vi "SplitLinesByDevice.vi"(8 "error in":errorcluster, 11 "Lines":tag[](array[tag])) -> (0 "error out":errorcluster, 1 "Num lines":i32, 2 "Original indices":i32[][](array[numeric]), 3 "Lines by device":string[](array[string]))   [LabVIEW 2015]
doc: "Splits the input lines into an array of lines where each array element is a flattened (comma-delimited string) list of devices belonging to a given channel.\n\nThe \"Original indices\" 2D array tells you how the new lines (being an array of lists) maps back to the original 1D indices."
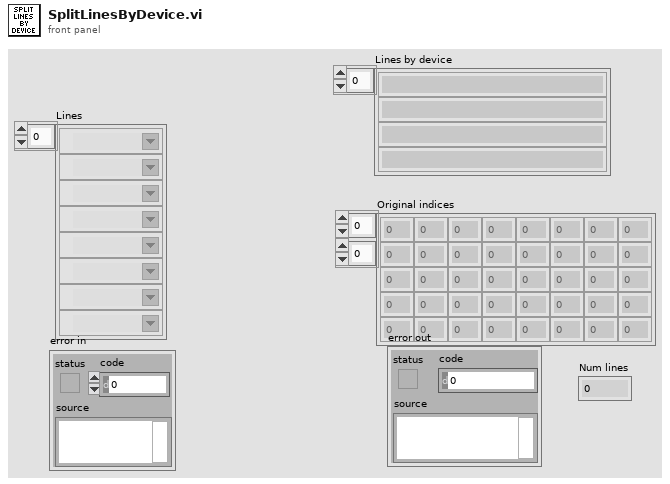
[diagram p1: front panel]
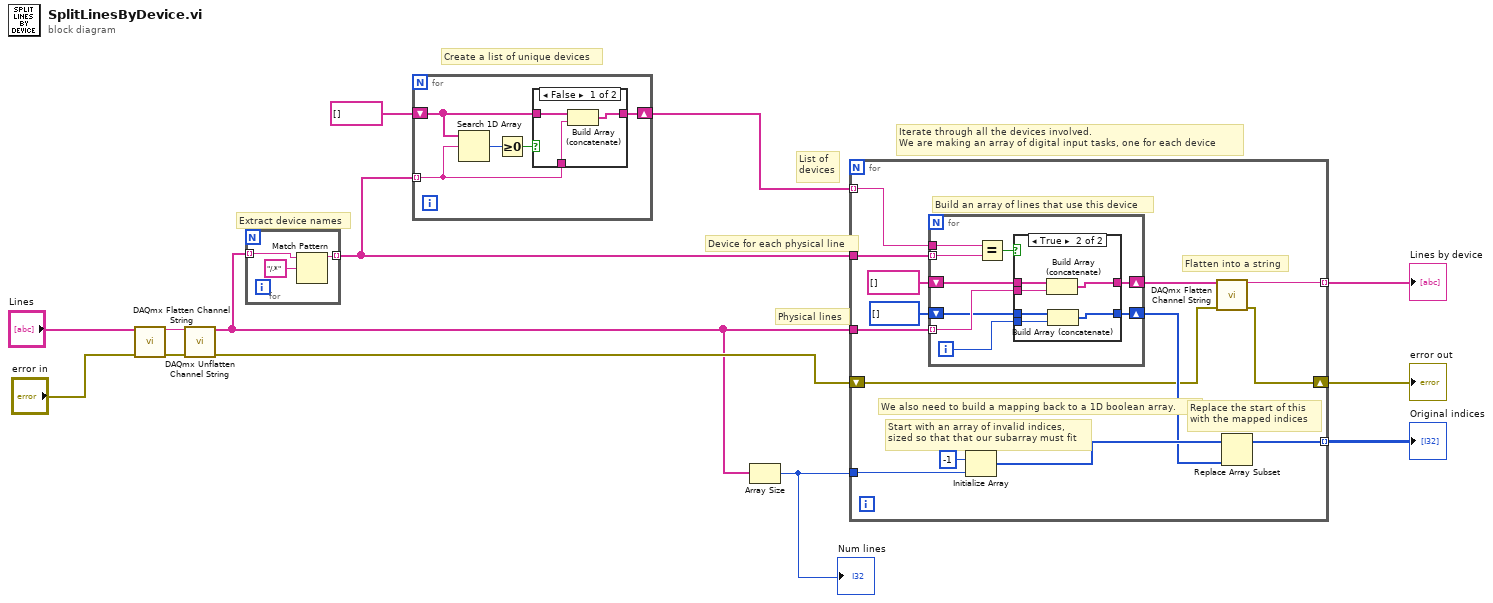
[diagram p0: block diagram]
diagram:
  # "Create a list of unique devices"
  # "Iterate through all the devices involved.\nWe are making an array of digital input tasks, one for each device"
  # "Device for each physical line"
  # "Extract device names"
  # "Physical lines"
  # "List of\ndevices"
  n1 = call <vilib>:"DAQmx Flatten Channel String.vi"("names in"="Lines", "error in"="error in") -> ("names out"=w12:string, "error out"=w6:errorcluster)  [unwired: 12 in]
  n2 = call <vilib>:"DAQmx Unflatten Channel String.vi"("names in"=w12, "error in"=w6) -> ("names out"=w1:string[], "error out"=w5:errorcluster)  [unwired: 12 in]
  n3 = for {
    tunnel: w1 -> [w16] mode=indexing
    tunnel: [w14] -> w10 mode=indexing
    n4 = Match Pattern(string=w16, regular expression="/.*") -> (before substring=w14:string)  [unwired: 1 in, 3 out]
  }
  n5 = for {
    tunnel: w10 -> [w18] mode=indexing
    shift-right: [w19] -> w8
    shift-left: string[] [] -> [w20]
    n6 = Search 1D Array(1D array=w20, element=w18) -> (index of element=w21:i32)  [unwired: 1 in]
    n7 = Greater Or Equal To 0?(x=w21) -> (x >= 0?=w17:bool)
    n8 = case shown="False" w17 {
      tunnel: w20 -> [w24 w25]
      tunnel: [w23 w25] -> w19
      tunnel: w18 -> [w22 _]
      frame False {
        n9 = Build Array (concatenate)(w24, w22) -> (w23:string[])
      }
      frame True {
      }
    }
  }
  n10 = Array Size(array=w1) -> (size(s)=w2:i32)
  "Num lines" <- w2
  n11 = for {
    tunnel: w1 -> [w35]
    tunnel: w10 -> [w39]
    tunnel: [w29] -> w3 mode=indexing
    tunnel: [w31] -> w11 mode=indexing
    tunnel: w8 -> [w30] mode=indexing
    shift-right: [w27] -> w4
    shift-left: w5 -> [w28]
    tunnel: w2 -> [w26]
    # "Replace the start of this\nwith the mapped indices"
    # "Start with an array of invalid indices,\nsized so that that our subarray must fit"
    # "We also need to build a mapping back to a 1D boolean array."
    # "Flatten into a string"
    # "Build an array of lines that use this device"
    n12 = for {
      tunnel: w39 -> [w40] mode=indexing
      tunnel: w35 -> [w47] mode=indexing
      shift-right: [w44] -> w36
      shift-left: string[] [] -> [w45]
      shift-right: [w42] -> w32
      shift-left: i32[] [] -> [w43]
      tunnel: w30 -> [w41]
      i -> [w46]
      n13 = Equal?(x=w41, y=w40) -> (x = y?=w48:bool)
      n14 = case shown="True" w48 {
        tunnel: w47 -> [_ w56]
        tunnel: w46 -> [_ w55]
        tunnel: w45 -> [w50 w54]
        tunnel: [w50 w53] -> w44
        tunnel: w43 -> [w49 w52]
        tunnel: [w49 w51] -> w42
        frame False {
        }
        frame True {
          n15 = Build Array (concatenate)(w54, w56) -> (w53:string[])
          n16 = Build Array (concatenate)(w52, w55) -> (w51:i32[])
        }
      }
    }
    n17 = Initialize Array(-1 ("element"), w26) -> (w33:i32[])
    n18 = call <vilib>:"DAQmx Flatten Channel String.vi"("names in"=w36, "error in"=w28) -> ("names out"=w29:string, "error out"=w27:errorcluster)  [unwired: 12 in]
    n19 = Replace Array Subset(array=w33, new element=w32) -> (w31:i32[])  [unwired: 1 in]
  }
  "Original indices" <- w11
  "error out" <- w4
  "Lines by device" <- w3
